vi "Align Velocity.vi"(4 "Period":i32, 5 "Translational Setpoints":dbl, 6 "AprilTag Pos":dbl, 7 "Deadband":dbl, 8 "Velocity Max":dbl=8.0, 9 "Acceleration Max":dbl=0.75) -> (0 "At Setpoint?":bool, 2 "Array size":i32, 3 "Velocity values":dbl[](array[numeric]))   [LabVIEW 2023]
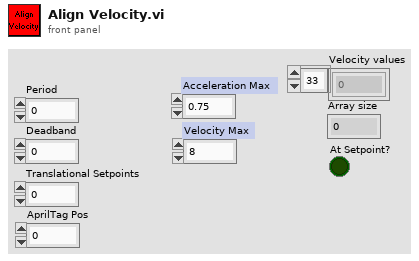
[diagram p1: front panel]
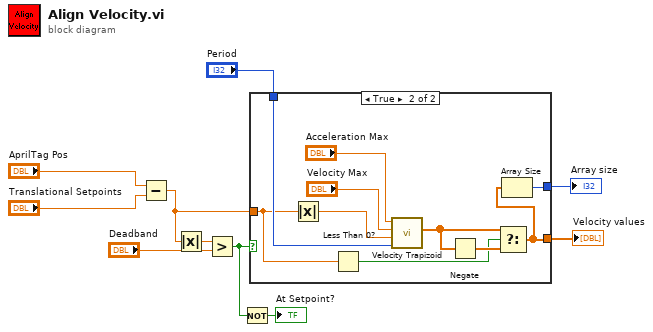
[diagram p0: block diagram]
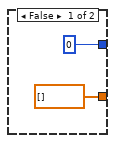
[diagram p2: hidden frame]
diagram:
  n1 = Subtract(x="AprilTag Pos", y="Translational Setpoints") -> (x-y=w2:dbl)
  n2 = Absolute Value(x=w2) -> (abs(x)=w1:dbl)
  n3 = Greater?(x=w1, y="Deadband") -> (0:w4:bool)
  n4 = Not(x=w4) -> (.not. x?=→"At Setpoint?":bool)
  n5 = case shown="True" w4 {
    tunnel: "Period" -> [_ w17]
    tunnel: [dbl[] [] ("Velocity values") w16] -> w5
    tunnel: [0 w15] -> w6
    tunnel: w2 -> [_ w14]
    frame False {
    }
    frame True {
      n6 = Absolute Value(x=w14) -> (abs(x)=w13:dbl)
      n7 = Less Than 0?(x=w14) -> (x < 0?=w18:bool)
      n8 = call "Velocity Trapizoid.vi"("Period"=w17, "Distance"=w13, "Velocity Max"="Velocity Max", "Acceleration Max"="Acceleration Max") -> ("Velocity values"=w20:dbl[])  [unwired: 6 in, 1 out]
      n9 = Negate(x=w20) -> (-x=w19:dbl[])
      n10 = Select(t=w20, s=w18, f=w19) -> (s? t:f=w16:dbl[])
      n11 = Array Size(array=w16) -> (size(s)=w15:i32)
    }
  }
  "Array size" <- w6
  "Velocity values" <- w5
